vi "Retrieve Conversion Factor from Excel.vi"(8 "error in (no error)":errorcluster, 10 "Row":u16, 11 "report in":refnum<class "NI_report.lvclass">) -> (0 "error out":errorcluster, 2 "Conversion factor":dbl, 3 "report out":refnum<class "NI_report.lvclass">)   [LabVIEW 2019]
doc: "For use with Tektronix Excel Data Reports\n\nReturns the conversion factor for the prefix in the units column of the given Row"
uses:
  <vilib>/Utility/NIReport.llb/NI_report.lvclass
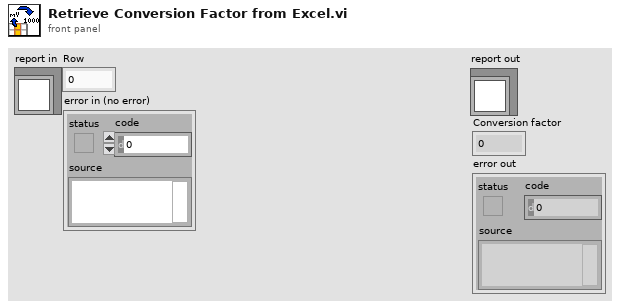
[diagram p1: front panel]
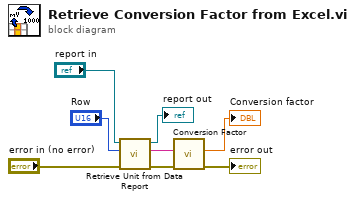
[diagram p0: block diagram]
diagram:
  n1 = call <userlib>:"Retrieve Unit from Data Report.vi"("error in (no error)"="error in (no error)", "Row"="Row", "report in"="report in") -> ("error out"=w2:errorcluster, "data"=w8:string, "report out"=→"report out":refnum<class "NI_report.lvclass">)  [unwired: 6 in]
  n2 = call <userlib>:"Conversion Factor.vi"("error in (no error)"=w2, "Unit"=w8) -> ("error out"=→"error out":errorcluster, "Conversion factor"=→"Conversion factor":dbl)  [unwired: 8 in]
